vi "RT Globals.vi"() -> ()   [LabVIEW 2019, in "Scan Engine Custom Device.lvlib"]
uses:
  Scan Engine Custom Device.lvlib
panel:
  in  "Cyclic Data Bandwidth Default":u32=40
  in  "PCL Sync?":bool
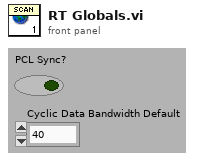
[diagram p1: front panel]
diagram:
